vi "Shared Variable Test.vi"() -> ()   [LabVIEW 2012]
panel:
  in  "Stop Button":bool
  in  "Boolean Control":bool
  out "Boolean Indicator":bool
  out "String Indicator":string
  in  "String Control":string
  in  "Knob":dbl(knob) scale=0.0..10.0
  out "Vertical Fill Slide":dbl(slide) scale=0.0..10.0
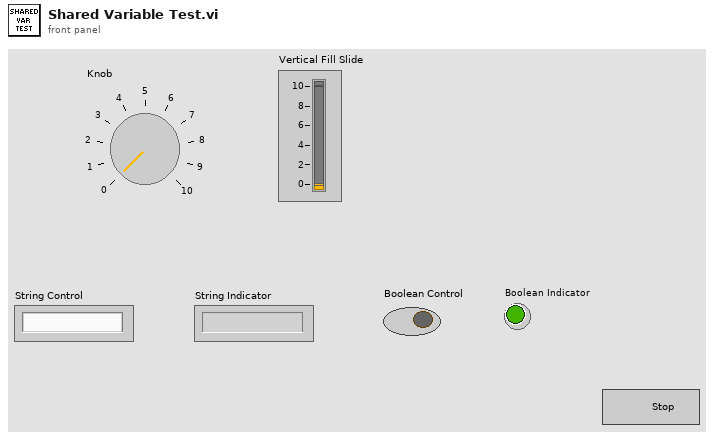
[diagram p1: front panel]
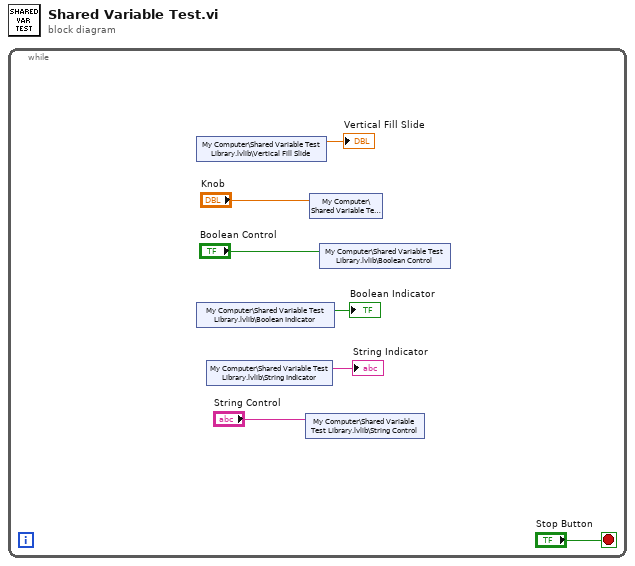
[diagram p0: block diagram]
diagram:
  n1 = while {
    stop <- "Stop Button" stop-if-true
    n2 = shared-variable "My Computer\\Shared Variable Test Library.lvlib\\Vertical Fill Slide"() -> (→"Vertical Fill Slide":dbl)  [unwired: 1 in, 1 out]
    n3 = shared-variable "My Computer\\Shared Variable Test Library.lvlib\\Boolean Indicator"() -> (→"Boolean Indicator":bool)  [unwired: 1 in, 1 out]
    n4 = shared-variable "My Computer\\Shared Variable Test Library.lvlib\\String Indicator"() -> (→"String Indicator":string)  [unwired: 1 in, 1 out]
    n5 = shared-variable "My Computer\\Shared Variable Test Library.lvlib\\String Control"("String Control") -> ()  [unwired: 1 in, 1 out]
    n6 = shared-variable "My Computer\\Shared Variable Test Library.lvlib\\Knob"("Knob") -> ()  [unwired: 1 in, 1 out]
    n7 = shared-variable "My Computer\\Shared Variable Test Library.lvlib\\Boolean Control"("Boolean Control") -> ()  [unwired: 1 in, 1 out]
  }
